vi "FPGA Interleaving.vi"() -> ()   [LabVIEW 2012]
uses:
  <vilib>/LabVIEW Targets/FPGA/cRIO/shared/nicrio_ModuleControls/nicrio_cRIO-9234_DataRatesRing2.ctl
  <vilib>/rvi/Emulation/niFpgaSctlEmulationGetInTimedLoop.vi
  <vilib>/rvi/Emulation/niFpgaSctlEmulationGlobalWrite.vi
  <vilib>/rvi/eio/common/nirviEmuTemplatePropertySet_noerrors.vi
  <vilib>/rvi/eio/common/nirviEmuTemplateMethod_errors.vi
  <vilib>/rvi/interface/RandomDataEmulation/nirviRandomDataFPGAFIFO.vi
  <vilib>/rvi/interface/RandomDataEmulation/niFpgaRandomDataHandleErrors.vi
  <vilib>/eio/EIOPropertyNode/EIOPropertyNode.xnode
  <vilib>/eio/EIONode/EIONode.xnode
  <vilib>/rvi/DataTransferAndStorage/Container/XNode/niFpgaContainer.xnode
  <vilib>/rvi/interface/RandomDataEmulation/nirviRandomDataFpgaReadWriteTemplate.vi
  <vilib>/rvi/eio/common/nirviEmuTemplatePropertyGet_errors.vi
  <vilib>/rvi/eio/common/nirviEmuTemplatePropertyGet_noerrors.vi
  <vilib>/rvi/eio/common/nirviEmuTemplatePropertySet_errors.vi
panel:
  in  "Data Rate":T1=1 items=["51.200 kS/s (NI 9234)"=1, "25.600 kS/s (NI 9234)"=2, "17.067 kS/s (NI 9234)"=3, "12.800 kS/s (NI 9234)"=4, "10.240 kS/s (NI 9234)"=5, "8.533 kS/s (NI 9234)"=6, "7.314 kS/s (NI 9234)"=7, "6.400 kS/s (NI 9234)"=8, "5.689 kS/s (NI 9234)"=9, "5.120 kS/s (NI 9234)"=10, "4.654 kS/s (NI 9234)"=11, "4.267 kS/s (NI 9234)"=12, "3.938 kS/s (NI 9234)"=13, "3.657 kS/s (NI 9234)"=14, "3.413 kS/s (NI 9234)"=15, "3.200 kS/s (NI 9234)"=16, "3.012 kS/s (NI 9234)"=17, "2.845 kS/s (NI 9234)"=18, "2.695 kS/s (NI 9234)"=19, "2.560 kS/s (NI 9234)"=20, "2.438 kS/s (NI 9234)"=21, "2.328 kS/s (NI 9234)"=22, "2.226 kS/s (NI 9234)"=23, "2.133 kS/s (NI 9234)"=24, "2.048 kS/s (NI 9234)"=25, "1.969 kS/s (NI 9234)"=26, "1.896 kS/s (NI 9234)"=27, "1.829 kS/s (NI 9234)"=28, "1.765 kS/s (NI 9234)"=29, "1.707 kS/s (NI 9234)"=30, "1.652 kS/s (NI 9234)"=31]
  in  "stop":bool
  in  "DMA Cleared?":bool
  out "Overflow?":bool
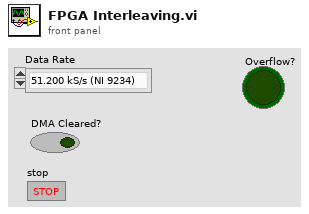
[diagram p1: front panel]
types:
  T1 = typedef "nicrio_cRIO-9234_DataRatesRing2.ctl" = u8
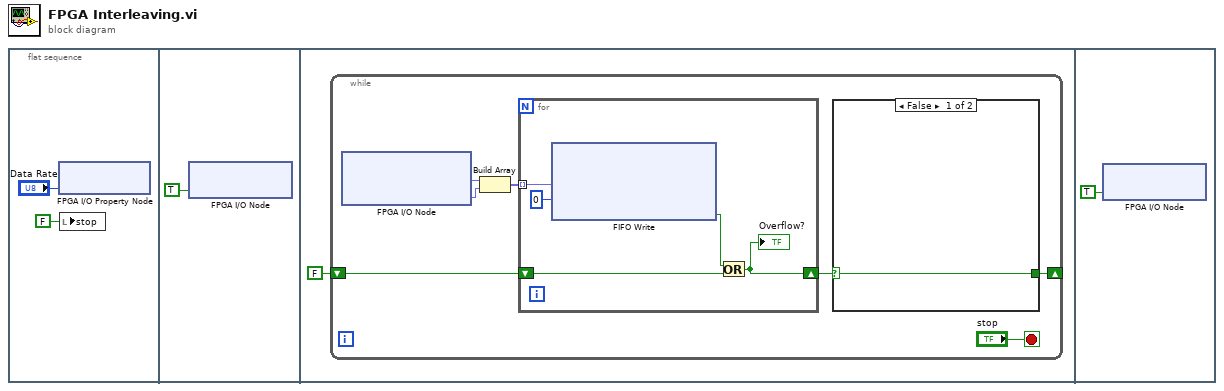
[diagram p0: block diagram]
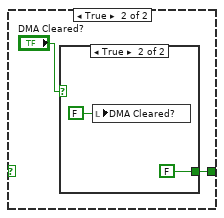
[diagram p2: hidden frame]
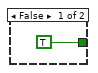
[diagram p3: hidden frame]
diagram:
  n1 = flat-sequence {
    frame #0 {
      n2 = xnode "FPGA I/O Property Node"("Data Rate"="Data Rate") -> ()  [unwired: 1 in, 1 out]
      n3 = local write "stop"(FALSE ("stop")) -> ()
    }
    frame #1 {
      n4 = xnode "FPGA I/O Node"("Mod2/Start"=TRUE) -> ()  [unwired: 1 in, 1 out]
    }
    frame #2 {
      n5 = while {
        shift-right: [w7] -> _
        shift-left: FALSE -> [w6]
        stop <- "stop" stop-if-true
        n6 = xnode "FPGA I/O Node"() -> ("Accelerometer 0"=w9:fxp<+/-,24,4>, "Accelerometer 1"=w10:fxp<+/-,24,4>)  [unwired: 2 in, 2 out]
        n7 = Build Array "Build Array"(w9, w10) -> (w11:fxp<+/-,24,4>[])
        n8 = for {
          tunnel: w11 -> [w21] mode=indexing
          shift-right: [w19] -> w8
          shift-left: w6 -> [w20]
          n9 = xnode "FIFO Write"("Element"=w21, "Timeout"=0) -> ("Timed Out?"=w22:bool)  [unwired: 1 in, 1 out]
          n10 = Or(x=w22, y=w20) -> (x .or. y?=w19:bool)
          "Overflow?" <- w19
        }
        n11 = case shown="False" w8 {
          selector: w8 -> [w12 _]
          tunnel: [w12 w13] -> w7
          frame False {
          }
          frame True {
            n12 = case shown="True" "DMA Cleared?" {
              tunnel: [TRUE FALSE] -> w13
              frame False {
              }
              frame True {
                n13 = local write "DMA Cleared?"(FALSE ("Reset")) -> ()
              }
            }
          }
        }
      }
    }
    frame #3 {
      n14 = xnode "FPGA I/O Node"("Mod2/Stop"=TRUE) -> ()  [unwired: 1 in, 1 out]
    }
  }
